vi "Status.vi"(8 "error in (no error)":errorcluster, 10 "Internal?":bool, 11 "Huber Settings":T1) -> (0 "error out":errorcluster, 1 "Connection Error":bool, 2 "Running":bool, 3 "Huber Settings":T1, 6 "Temperature":i32)   [LabVIEW 2018, in "Huber Unistat 410 TCU.lvlib"]
uses:
  Huber Unistat 410 TCU.lvlib
  Huber Unistat 410 Settings.ctl
  <vilib>/regexp/Match Regular Expression.xnode
panel:
  out "substring":string
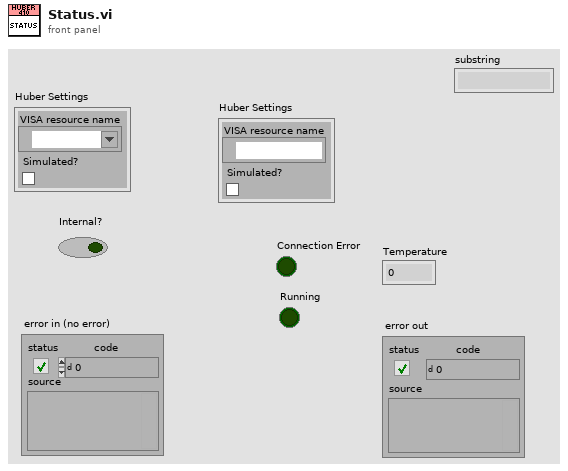
[diagram p1: front panel]
types:
  T1 = typedef "Huber Unistat 410 TCU.lvlib/Huber Unistat 410 Settings.ctl" = cluster{"VISA resource name":refnum<visa-resource-name>, "Simulated?":bool}
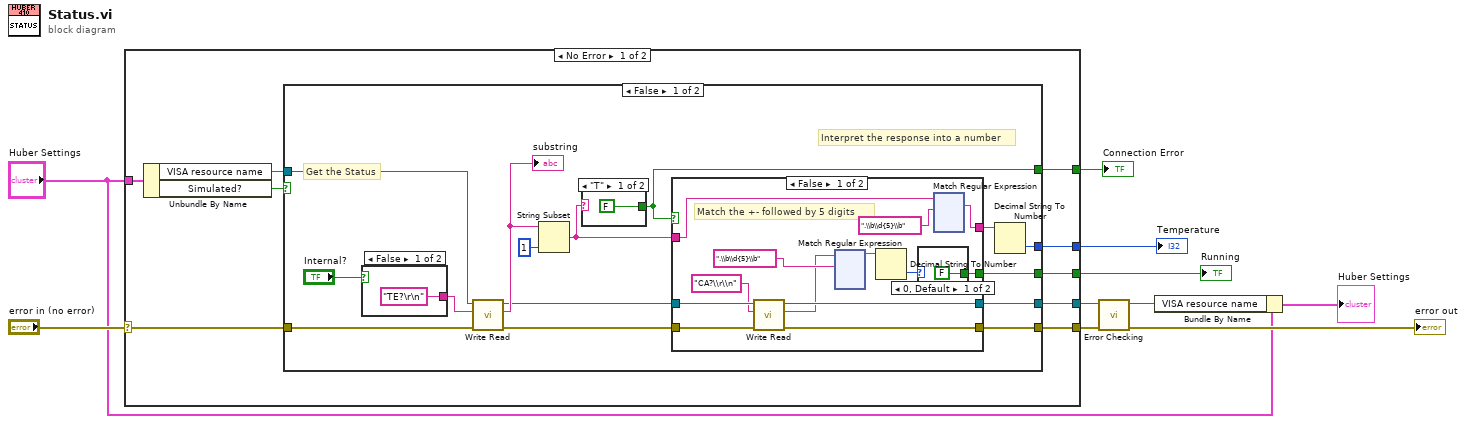
[diagram p0: block diagram]
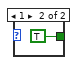
[diagram p2: hidden frame]
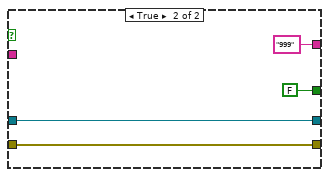
[diagram p3: hidden frame]
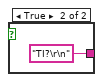
[diagram p4: hidden frame]
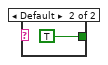
[diagram p5: hidden frame]
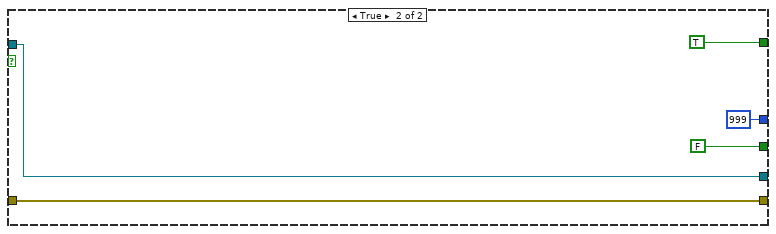
[diagram p6: hidden frame]
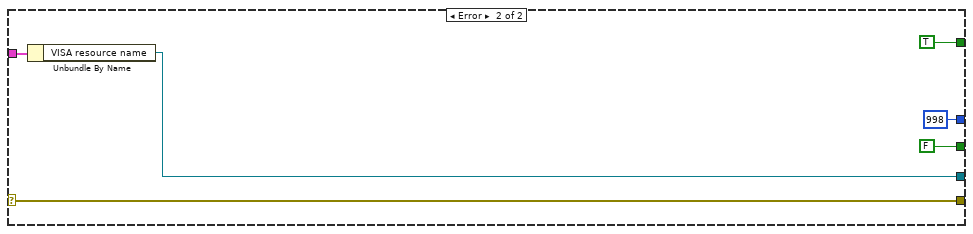
[diagram p7: hidden frame]
diagram:
  n1 = case shown="No Error" "error in (no error)" {
    selector: "error in (no error)" -> [w19 w296]
    tunnel: "Huber Settings" -> [w17 w295]
    tunnel: [w18 w296] -> w8
    tunnel: [w15 w294] -> w9
    tunnel: [w13 TRUE] -> w3
    tunnel: [w12 FALSE] -> w2
    tunnel: [w11 998] -> w1
    frame No Error {
      n2 = Unbundle By Name(w17) -> ("VISA resource name"=w16:refnum<visa-resource-name>, "Simulated?"=w14:bool)
      n3 = case shown="False" w14 {
        tunnel: w19 -> [w31 w290]
        tunnel: [w25 w290] -> w18
        tunnel: [w22 w289] -> w15
        tunnel: w16 -> [w32 w289]
        tunnel: [w27 TRUE] -> w13
        tunnel: [w23 FALSE] -> w12
        tunnel: [w21 999] -> w11
        frame False {
          # "Interpret the response into a number"
          # "Get the Status"
          n4 = case shown="False" "Internal?" {
            tunnel: ["TE?\r\n" ("string") "TI?\r\n" ("string")] -> w34
            frame False {
            }
            frame True {
            }
          }
          n5 = call "Write Read.vi"("error in (no error)"=w31, "write string"=w34, "VISA Refnum in"=w32) -> ("error out"=w26:errorcluster, "read string"=w30:string, "VISA Refnum out"=w24:refnum<visa-resource-name>)  [unwired: 6 in]
          "substring" <- w30
          n6 = String Subset(string=w30, length (rest)=1 ("length (rest)")) -> (substring=w28:string)  [unwired: 1 in]
          n7 = case shown="\"T\"" w28 {
            tunnel: [FALSE TRUE] -> w27
            frame "T" {
            }
            frame Default {
            }
          }
          n8 = case shown="False" w27 {
            tunnel: w28 -> [w47 _]
            tunnel: [w46 "999" ("whole match")] -> w20
            tunnel: w26 -> [w40 w280]
            tunnel: [w39 w280] -> w25
            tunnel: w24 -> [w42 w278]
            tunnel: [w44 FALSE] -> w23
            tunnel: [w38 w278] -> w22
            frame False {
              # "Match the +- followed by 5 digits"
              n9 = call "Write Read.vi"("error in (no error)"=w40, "write string"="CA?\\r\\n" ("string"), "VISA Refnum in"=w42) -> ("error out"=w39:errorcluster, "read string"=w36:string, "VISA Refnum out"=w38:refnum<visa-resource-name>)  [unwired: 6 in]
              n10 = xnode "Match Regular Expression"("input string"=w36, "regular expression"=".\\b\\d{5}\\b") -> ("whole match"=w35:string)  [unwired: 4 in, 4 out]
              n11 = Decimal String To Number(string=w35) -> (number=w43:i32)  [unwired: 2 in, 1 out]
              n12 = case shown="0, Default" w43 {
                tunnel: [FALSE TRUE] -> w44
                frame 0, Default {
                }
                frame 1 {
                }
              }
              n13 = xnode "Match Regular Expression"("input string"=w47, "regular expression"=".\\b\\d{5}\\b") -> ("whole match"=w46:string)  [unwired: 4 in, 4 out]
            }
            frame True {
            }
          }
          n14 = Decimal String To Number(string=w20) -> (number=w21:i32)  [unwired: 2 in, 1 out]
        }
        frame True {
        }
      }
    }
    frame Error {
      n15 = Unbundle By Name(w295) -> ("VISA resource name"=w294:refnum<visa-resource-name>)
    }
  }
  "Connection Error" <- w3
  "Running" <- w2
  "Temperature" <- w1
  n16 = call "Error Checking.vi"("error in (no error)"=w8, "VISA resource name"=w9) -> ("error out"=→"error out":errorcluster, "VISA resource name"=w6:refnum<visa-resource-name>)  [unwired: 7 in, 1 out]
  n17 = Bundle By Name(cluster="Huber Settings", "VISA resource name"=w6) -> (→"Huber Settings":T1)
